vi "HP8753 Trigger_1.0.0.0.vi"(1 "trigger source (0 : ext trig off)":u16(ring) items=["external trigger off", "external trigger on sweep", "external trigger on point", "manual trigger on point"], 3 "error in (no error)":errorcluster, 4 "number of groups":u16=16 min=1 max=999, 5 "trigger (1 : single)":u16(ring) items=["hold", "single", "number of groups", "continuous"], 6 "VISA session":refnum<visa-resource-name>) -> (0 "error out":errorcluster, 2 "dup VISA session":refnum<visa-resource-name>)   [LabVIEW 2018]
doc: "This VI for the HP8753B Network Analyzer sets up the triggering.\n\nNOTE: If Manual trigger is selected in the trigger source control, then only the the continuous trigger type is valid, therefore the continuous trigger type is automatically sent with the manual trigger selection, and the trigger type selection is ignored."
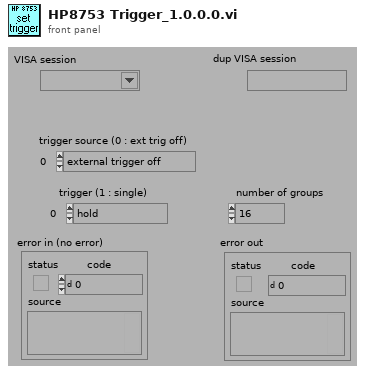
[diagram p1: front panel]
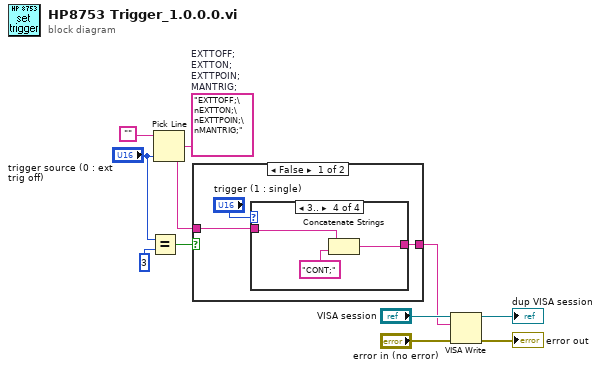
[diagram p0: block diagram]
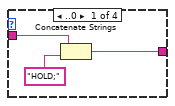
[diagram p2: hidden frame]
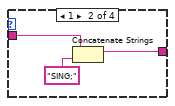
[diagram p3: hidden frame]
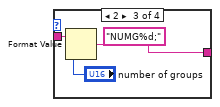
[diagram p4: hidden frame]
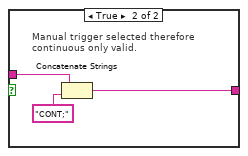
[diagram p5: hidden frame]
diagram:
  w9 = "EXTTOFF;\nEXTTON;\nEXTTPOIN;\nMANTRIG;"  # EXTTOFF; EXTTON; EXTTPOIN; MANTRIG;
  n1 = Equal?(x="trigger source (0 : ext trig off)", y=3) -> (x = y?=w3:bool)
  n2 = Pick Line(string ("")="", multi-line string=w9, line index="trigger source (0 : ext trig off)") -> (output string=w2:string)
  n3 = case shown="False" w3 {
    tunnel: w2 -> [w13 w29]
    tunnel: [w12 w28] -> w1
    frame False {
      n4 = case shown="3.." "trigger (1 : single)" {
        tunnel: [w15 w20 w22 w25] -> w12
        tunnel: w13 -> [w17 w18 w21 w26]
        frame ..0 {
          n5 = Concatenate Strings(w17, "HOLD;") -> (w15:string)
        }
        frame 1 {
          n6 = Concatenate Strings(w18, "SING;") -> (w20:string)
        }
        frame 2 {
          n7 = Format Value(string ("")=w21, format string="NUMG%d;", value (0)="number of groups") -> (output string=w22:string)
        }
        frame 3.. {
          n8 = Concatenate Strings(w26, "CONT;") -> (w25:string)
        }
      }
    }
    frame True {
      # "Manual trigger selected therefore\ncontinuous only valid."
      n9 = Concatenate Strings(w29, "CONT;") -> (w28:string)
    }
  }
  n10 = VISA Write(VISA resource name="VISA session", write buffer=w1, error in (no error)="error in (no error)") -> (VISA resource name out=→"dup VISA session":refnum<visa-resource-name>, error out=→"error out":errorcluster)  [unwired: 1 out]
